vi "CTRE_ErrorHandle.vi"(8 "error in":errorcluster, 10 "origin":string, 11 "code":i32) -> (0 "error out":errorcluster)   [LabVIEW 2016]
uses:
  <vilib>/Utility/error.llb/whitespace.ctl
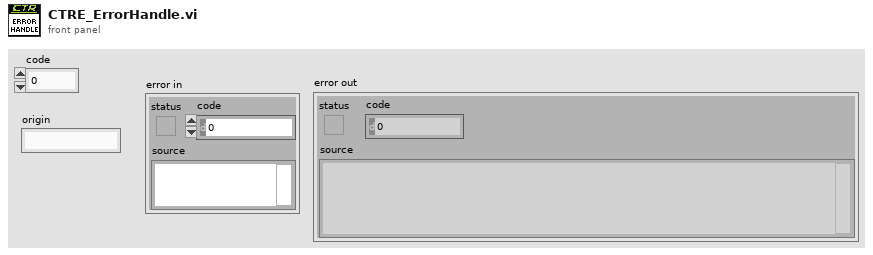
[diagram p1: front panel]
types:
  T1 = typedef "whitespace.ctl" = u16
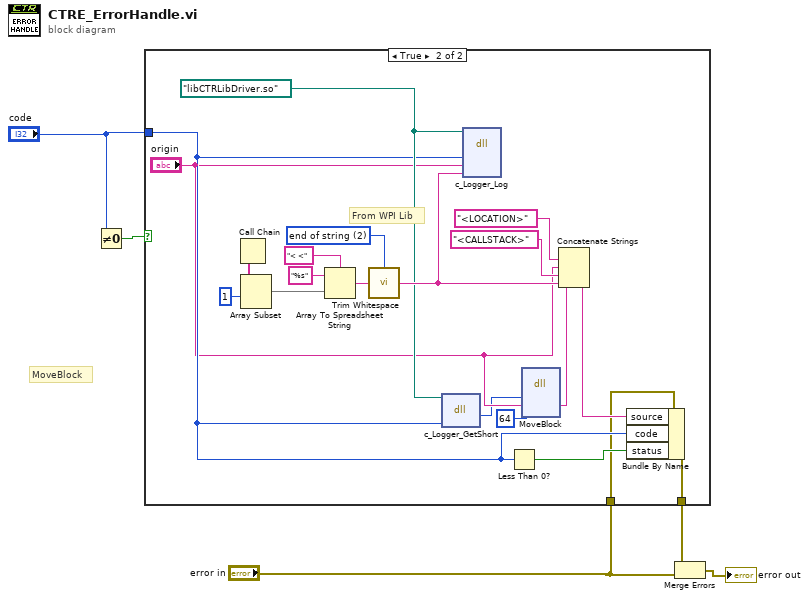
[diagram p0: block diagram]
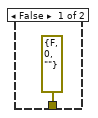
[diagram p2: hidden frame]
diagram:
  # "MoveBlock"
  n1 = Not Equal To 0?(x="code") -> (x != 0?=w4:bool)
  n2 = case shown="True" w4 {
    tunnel: "code" -> [_ w14]
    tunnel: [errorcluster {"status"=FALSE, "code"=0, "source"=""} ("error in") w12] -> w2
    tunnel: "error in" -> [_ w11]
    frame False {
    }
    frame True {
      w23 = T1 2 items=["both", "start of string", "end of string"] ("location (both)")
      w16 = path "libCTRLibDriver.so" ("path in")
      # "From WPI Lib"
      n3 = Call Chain() -> (call chain=w19:string[])
      n4 = Array Subset(array=w19, index=1) -> (w20:string[])  [unwired: 1 in]
      n5 = Array To Spreadsheet String(delimiter (Tab)="< <", array=w20, 3:"%s" ("format string")) -> (spreadsheet string=w24:string)
      n6 = call <vilib>:"Trim Whitespace.vi"("string"=w24, "location (both)"=w23) -> ("trimmed string"=w17:string)
      n7 = dll-call lib="?" fn="c_Logger_GetShort"(path in=w16, "CTRCode"=w14) -> ("return type"=w7:i64)  [unwired: 3 in, 2 out]
      n8 = dll-call lib="?" fn="c_Logger_Log"(path in=w16, "CTRCode"=w14, "origin"="origin", "stacktrace"=w17) -> ()  [unwired: 6 in, 2 out]
      n9 = Less Than 0?(x=w14) -> (x < 0?=w15:bool)
      n10 = dll-call lib="LabVIEW" fn="MoveBlock"("Address (Pointer)"=w7, "Destination"="origin", "Size"=64) -> ("Destination"=w9:string)  [unwired: 6 in, 2 out]
      n11 = Concatenate Strings(w9, "<LOCATION>" ("string"), "origin", "<CALLSTACK>" ("string"), w17) -> (w13:string)
      n12 = Bundle By Name(cluster=w11, "source"=w13, "code"=w14, "status"=w15) -> (w12:errorcluster)
    }
  }
  n13 = Merge Errors(w2, "error in") -> (→"error out":errorcluster)
